vi "Sub_secular_solver.vi"(0 "Eigenvalues":dbl[](array[numeric]), 5 "Transpose Eigenvectors":dbl[](array[numeric]), 7 "Empty Solution Array":dbl[](array[numeric]), 9 "Inverse Delta in Stiffness":dbl, 11 "Total Modes":i32, 12 "Total Corrections":i32=1) -> (4 "New Eigenvalues":dbl[](array[numeric]))   [LabVIEW 2021]
panel:
  # "Seclular solver"
  # "Documentation:  ipsum lorem"
  # "Inputs"
  # "Solution Parameters"
  # "Outputs"
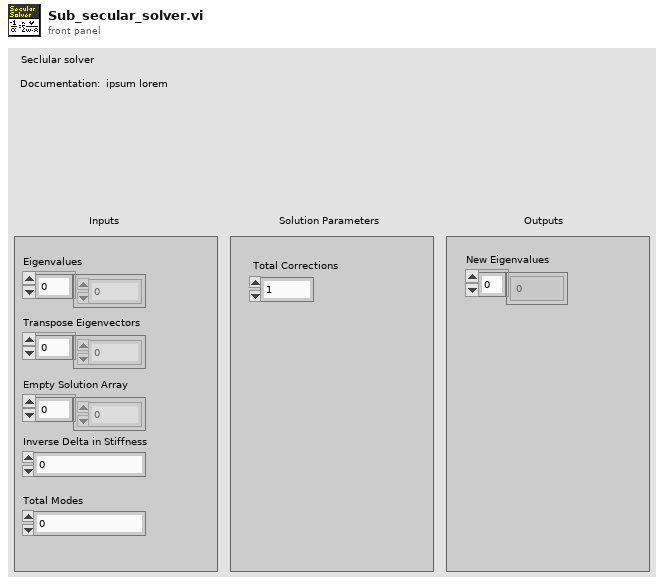
[diagram p1: front panel]
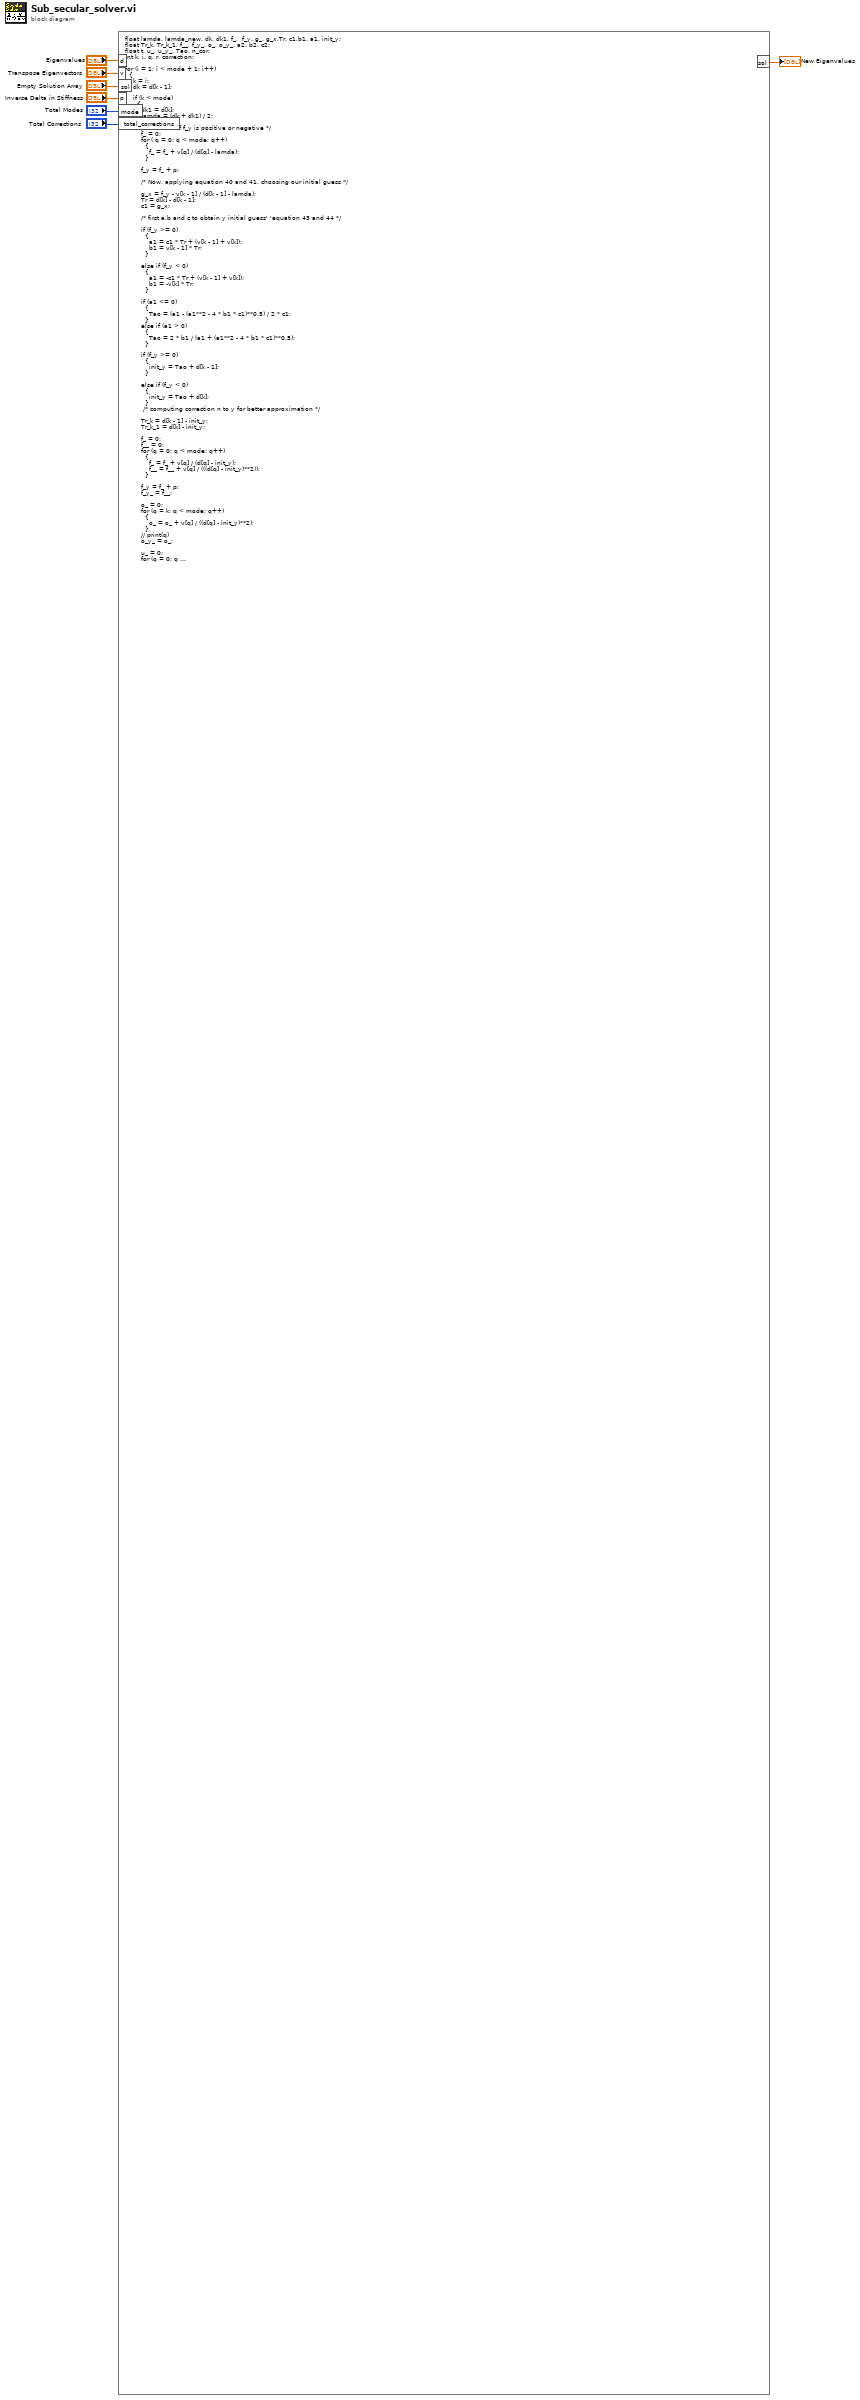
[diagram p0: block diagram]
diagram:
  n1 = formula code="float lamda, lamda_new, dk, dk1, f_,  f_y, g_, g_x,Tr, c1,b1, a1, init_y;\nfloat Tr_k, Tr_k_1, f__, f_y_, o_, o_y_, a2, b2, c2;\nfloat t, u_, u_y_, Tao, n_cor;\nint k, i, q, r, correction;\n\nfor (i = 1; i < mode + 1; i++)\n  {\n    k = i;\n    dk = d[k - 1];\n\n    if (k < mode)\n      {\n        dk1 = d[k];\n        lamda = (dk + dk1) / 2;\n\n        /* To check if f_y is positive or negative */\n        f_ = 0;\n        for ( q = 0; q < mode; q++)\n          {\n            f_ = f_ + v[q] / (d[q] - lamda);\n          }\n\n        f_y = f_ + p;\n\n        /* Now, applying equation 40 and 41, choosing our initial guess */\n\n        g_x = f_y - v[k - 1] / (d[k - 1] - lamda);\n        Tr = d[k] - d[k - 1];\n        c1 = g_x;\n\n        /* first a,b and c to obtain y initial guess' 'equation 43 and 44 */\n\n        if (f_y >= 0)\n          {\n            a1 = c1 * Tr + (v[k - 1] + v[k]);\n            b1 = v[k - 1] * Tr;\n          }\n\n        else if (f_y < 0)\n          {\n            a1 = -c1 * Tr + (v[k - 1] + v[k]);\n            b1 = -v[k] * Tr;\n          }\n\n        if (a1 <= 0)\n          {\n            Tao = (a1 - (a1**2 - 4 * b1 * c1)**0.5) / 2 * c1;\n          }\n        else if (a1 > 0)\n          {\n            Tao = 2 * b1 / (a1 + (a1**2 - 4 * b1 * c1)**0.5);\n          }\n\n        if (f_y >= 0)\n          {\n            init_y = Tao + d[k - 1];\n          }\n\n        else if (f_y < 0)\n          {\n            init_y = Tao + d[k];\n          }\n         /* computing correction n to y for better approximation */\n\n        Tr_k = d[k - 1] - init_y;\n        Tr_k_1 = d[k] - init_y;\n\n        f_ = 0;\n        f__ = 0;\n        for (q = 0; q < mode; q++)\n          {\n            f_ = f_ + v[q] / (d[q] - init_y);\n            f__ = f__ + v[q] / (((d[q] - init_y)**2));\n          }\n\n        f_y = f_ + p;\n        f_y_ = f__;\n\n        o_ = 0;\n        for (q = k; q < mode; q++)\n          {\n            o_ = o_ + v[q] / ((d[q] - init_y)**2);\n          }\n        // print(q)\n        o_y_ = o_;\n\n        u_ = 0;\n        for (q = 0; q < mode; q++)\n          {\n            u_ = u_ + v[q] / ((d[q] - init_y)**2);\n          }\n        // print(q)\n\n        u_y_ = u_;\n        /*'second a, b and c for final correction' */\n\n        a2 = (Tr_k + Tr_k_1) * f_y - Tr_k * Tr_k_1 * f_y_;\n        b2 = Tr_k * Tr_k_1 * f_y;\n\n        if (f_y >= 0)\n          {\n            c2 = f_y - Tr_k_1 * f_y_ - u_y_ * (d[k - 1] - d[k]);\n          }\n\n        else if (f_y < 0)\n          {\n            c2 = f_y - Tr_k * f_y_ - o_y_ * (d[k] - d[k - 1]);\n          }\n\n        if (a2 <= 0)\n          {\n            n_cor = (a2 - (a2**2 - 4 * b2 * c2)**0.5) / 2 * c2;\n          }\n\n        else if (a2 > 0)\n          {\n            n_cor = 2 * b2 / (a2 + (a2**2 - 4 * b2 * c2)**0.5);\n          }\n\n        lamda_new = init_y + n_cor;\n        /*computing second correction n to y for better approximation */\n        // init_y = lamda_new;\n\n        sol[k - 1] = lamda_new;\n      }\n\n    else if (k == mode)\n      {\n        t = 0;\n        for (r = 0; r < mode; r++)\n          {\n            t = t + (v[r]**2);\n          }\n\n        float d6;\n\n        d6 = d[k - 1] + t / p;\n\n        lamda = (d6 + d[k - 1]) / 2;\n\n        //'To check if f_y is positive or negative'\n\n        f_ = 0;\n        for( q = 0; q < mode; q++)\n          {\n            f_ = f_ + v[q] / (d[q] - lamda);\n          }\n\n        f_y = f_ + p;\n\n        //'Now, applying equation 40 and 41, choosing our initial guess'\n        /*g_ = 0;\n           for( q = 0; q<n; q++)\n           {\n           g_ = g_ + v[q]/(d[q]-lamda);\n           }\n\n           g_x = g_ + p; */\n\n        g_x = f_y - v[k - 1] / (d[k - 1] - lamda);\n        Tr = d[k - 1] - d[k - 2];\n        c1 = g_x;\n\n        //'first a,b and c to obtain y initial guess' 'equation 43 and 44'\n        if (f_y <= 0)\n          {\n            a1 = c1 * Tr + (v[k - 2] + v[k - 1]);\n            b1 = v[k - 1] * Tr;\n          }\n\n        else if (f_y > 0)\n          {\n            a1 = -c1 * Tr + (v[k - 2] + v[k - 1]);\n            b1 = -v[k - 1] * Tr;\n          }\n\n        if (a1 <= 0)\n          {\n            Tao = (a1 + (a1**2 - 4 * b1 * c1)**0.5) / 2 * c1;\n          }\n\n        else if (a1 > 0)\n          {\n            Tao = 2 * b1 / (a1 - (a1**2 - 4 * b1 * c1)**0.5);\n          }\n\n        init_y = Tao + d[k - 1];\n\n        //'computing correction n to y for better approximation'\n        for (correction = 1; correction < total_corrections; correction++)\n          {\n\n            Tr_k = d[k - 1] - init_y;\n            Tr_k_1 = d6 - init_y;\n\n            f_ = 0;\n            f__ = 0;\n            for (q = 0; q < mode; q++)\n              {\n                f_ = f_ + v[q] / (d[q] - init_y);\n                f__ = f__ + v[q] / ((d[q] - init_y)**2);\n              }\n\n            f_y = f_ + p;\n            f_y_ = f__;\n\n            u_ = 0;\n            for (q = 0; q < mode; q++)\n              {\n                u_ = u_ + v[q] / ((d[q] - init_y)**2);\n              }\n\n            u_y_ = u_;\n            //'second a, b and c for final correction'\n\n            a2 = (Tr_k + Tr_k_1) * f_y - Tr_k * Tr_k_1 * f_y_;\n            b2 = Tr_k * Tr_k_1 * f_y;\n            c2 = f_y - Tr_k * u_y_ - (v[k - 1] / Tr_k_1);\n\n            if (a2 <= 0)\n              {\n                n_cor = (a2 - (a2**2 - 4 * b2 * c2)**0.5) / 2 * c2;\n              }\n\n            else if (a2 > 0)\n              {\n                n_cor = 2 * b2 / (a2 + (a2**2 - 4 * b2 * c2)**0.5);\n              }\n\n            lamda_new = init_y + n_cor;\n            init_y = lamda_new;\n          }\n        sol[mode - 1] = lamda_new;\n      }\n  }"("d"="Eigenvalues", "v"="Transpose Eigenvectors", "p"="Inverse Delta in Stiffness", "mode"="Total Modes", "sol"="Empty Solution Array", "total_corrections"="Total Corrections") -> ("sol"=→"New Eigenvalues":dbl[])
